vi "Flash APL Example.vi"(0 "GEA Inputs":T1 {"Destination" format="%.0x"; "Source" format="%.0x"}, 2 "Force Update?":bool, 7 "APL Path":path, 11 "Error In":errorcluster, 12 "Broadcast":bool=TRUE) -> (4 "Result":i32(ring) items=["ImageRejected", "BoardNotFound", "UnableToGetGeaConfiguration", "WriteToFlashNotAllowed", "ImageDownloadedSuccessfully", "ImagePresent", "WriteToFlashFailed", "EraseFailed", "CrcFailed"], 6 "Pass/Fail":bool, 8 "Report Text":string, 15 "Error Out":errorcluster)   [LabVIEW 2016]
doc: "This standalone example will flash an APL file to the board specified."
uses:
  LabVIEW_GEA2_Toolkit.lvlibp/type defs/Source_Destination.ctl
  LabVIEW_GEA2_Toolkit.lvlibp
panel:
  in  "Reset Board?":bool=TRUE
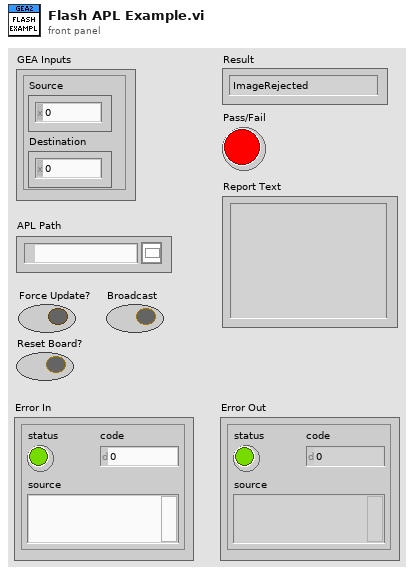
[diagram p1: front panel]
types:
  T1 = typedef "LabVIEW_GEA2_Toolkit.lvlibp/Source_Destination.ctl" = cluster{"Source":u8, "Destination":u8}
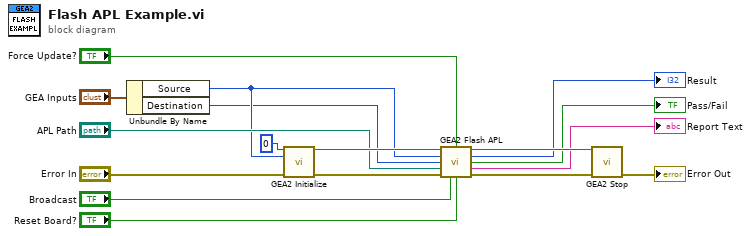
[diagram p0: block diagram]
diagram:
  n1 = Unbundle By Name("GEA Inputs") -> ("Source"=w7:u8, "Destination"=w6:u8)
  n2 = call "GEA2 Initialize.vi"("Board Index"=0, "Source Address"=w7, "error in"="Error In") -> ("GEA2 Reference Out"=w17:refnum<k24>, "error out"=w16:errorcluster)  [unwired: 10 in, 1 out]
  n3 = call "GEA2 Flash APL.vi"("GEA2 Reference In"=w17, "Force Update?"="Force Update?", "Source Address"=w7, "Destination Address"=w6, "File Path"="APL Path", "Error In"=w16, "Broadcast"="Broadcast", "Reset?"="Reset Board?") -> ("GEA2 Reference Out"=w14:refnum<k24>, "Result"=→"Result":i32, "Pass/Fail"=→"Pass/Fail":bool, "Report Text"=→"Report Text":string, "Error Out"=w13:errorcluster)  [unwired: 3 in]
  n4 = call "GEA2 Stop.vi"("GEA2 Reference In"=w14, "Error In"=w13) -> ("Error Out"=→"Error Out":errorcluster)  [unwired: 13 in]
